vi "GetConfigurationBasePath.vi"(8 "error in (no error)":errorcluster, 11 "reference in":refnum<class "IApplicationConfiguration.lvclass">) -> (0 "error out":errorcluster, 1 "ApplicationBasePath":path, 3 "reference out":refnum<class "IApplicationConfiguration.lvclass">)   [LabVIEW 2021, in "IApplicationConfiguration.lvclass"]
uses:
  IApplicationConfiguration.lvclass
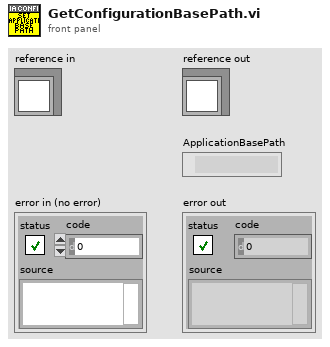
[diagram p1: front panel]
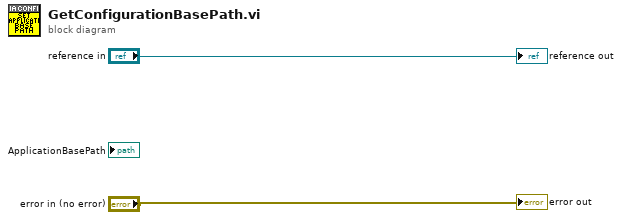
[diagram p0: block diagram]
diagram:
  "error out" <- "error in (no error)"
  "reference out" <- "reference in"
